vi "Create a New Run (typed).vi"(7 "xwpfRun Type":refnum<class "xwpfRun.lvclass">, 8 "error in (no error)":errorcluster, 10 "Text":string, 11 "Run Ref":refnum<k24>) -> (0 "error out":errorcluster, 3 "xwpfRun out":refnum<class "xwpfRun.lvclass">)   [LabVIEW 2017, in "Word_Specific.lvlib" / "xwpfRun.lvclass"]
uses:
  xwpfRun.lvclass
  C:/Users/Neo/Desktop/Dev_Tools_BR/LabVIEW_NPOI/lib/NPOI 2.1.1/NPOI.OOXML.dll
  lib/NPOI 2.1.1/NPOI.OOXML.dll
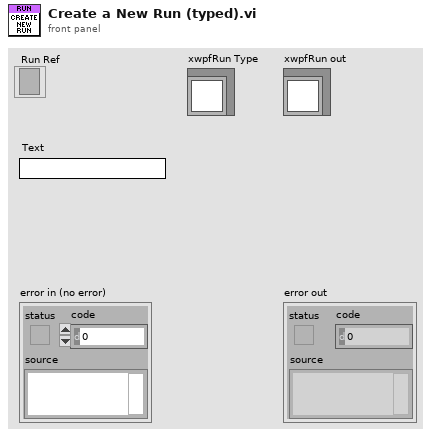
[diagram p1: front panel]
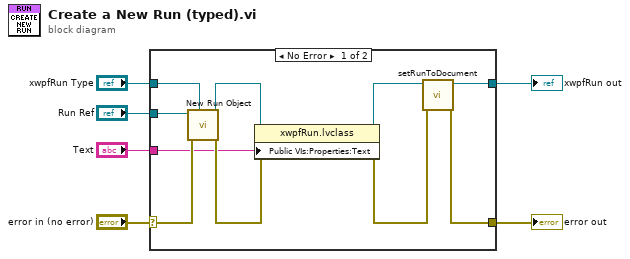
[diagram p0: block diagram]
diagram:
  n1 = case shown="No Error" "error in (no error)" {
    selector: "error in (no error)" -> [w10 w18]
    tunnel: [w9 w18] -> w5
    tunnel: [w12 w17] -> w3
    tunnel: "xwpfRun Type" -> [w16 w17]
    tunnel: "Run Ref" -> [w15 _]
    tunnel: "Text" -> [w7 _]
    frame No Error {
      n2 = call "New Run Object.vi"("xwpfRun Type"=w16, "error in (no error)"=w10, "Run Ref"=w15) -> ("error out"=w14:errorcluster, "xwpfRun out"=w13:refnum<class "xwpfRun.lvclass">)  [unwired: 7 in]
      n3 = property class="xwpfRun.lvclass"(reference=w13, error in=w14, "Public VIs:Properties:Text"=w7) -> (reference out=w11:refnum<class "xwpfRun.lvclass">, error out=w8:errorcluster)
      n4 = call-dynamic "setRunToDocument.vi"("error in (no error)"=w8, "xwpfRun in"=w11) -> ("error out"=w9:errorcluster, "xwpfRun out"=w12:refnum<class "xwpfRun.lvclass">)  [unwired: 8 in]
    }
    frame Error {
    }
  }
  "error out" <- w5
  "xwpfRun out" <- w3
